vi "Set Double.vi"(8 "error in":errorcluster, 9 "value":dbl, 10 "variable name":string, 11 "GOLPI ref. in":T1={"pipe handle"={"lv_proc.dll file path"=path "", "process instance handle"=[], "debug mode"=FALSE, "debug data"=[]}, "fast read timeout [ms]"=500, "fast read settle time [ms]"=10, "fast read to multiple [ms]"=1, "max elements per input line"=100, "slow read timeout [ms]"=5000, "stdin double format specifier"="", "max elements per stdout output column"=100, "console mode bitstream"=FALSE, "bitstream first read timeout [ms]"=1000, "bitstream read timeout [ms]"=50, "struct transfer possible"=FALSE, "matlab mode"=FALSE}) -> (0 "error out":errorcluster, 3 "GOLPI ref. out":T1={"pipe handle"={"lv_proc.dll file path"=path "", "process instance handle"=[], "debug mode"=FALSE, "debug data"=[]}, "fast read timeout [ms]"=500, "fast read settle time [ms]"=10, "fast read to multiple [ms]"=1, "max elements per input line"=100, "slow read timeout [ms]"=5000, "stdin double format specifier"="", "max elements per stdout output column"=100, "console mode bitstream"=FALSE, "bitstream first read timeout [ms]"=1000, "bitstream read timeout [ms]"=50, "struct transfer possible"=FALSE, "matlab mode"=FALSE})   [LabVIEW 2020, in "GOLPI library.lvlib"]
doc: "Part of polymorph Set Variable.vi"
uses:
  GOLPI library.lvlib
  GOLPI reference Type Def.ctl
  Pipe Handle.ctl
  LV Process library.lvlib
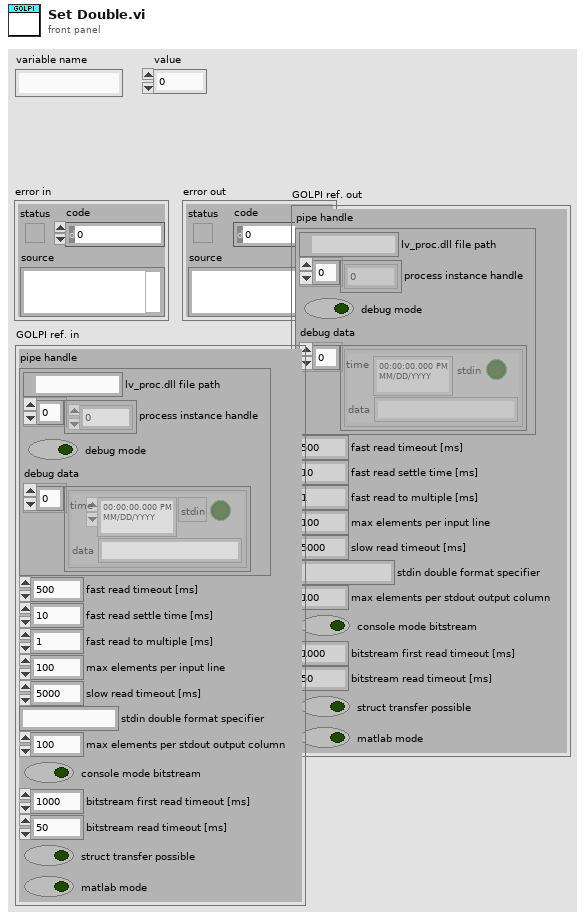
[diagram p1: front panel]
types:
  T1 = typedef "GOLPI library.lvlib/GOLPI reference Type Def.ctl" = cluster{"pipe handle":T2, "fast read timeout [ms]":u32, "fast read settle time [ms]":u32, "fast read to multiple [ms]":u32, "max elements per input line":u32, "slow read timeout [ms]":u32, "stdin double format specifier":string, "max elements per stdout output column":u32, "console mode bitstream":bool, "bitstream first read timeout [ms]":u32, "bitstream read timeout [ms]":u32, "struct transfer possible":bool, "matlab mode":bool}
  T2 = typedef "LV Process library.lvlib/Pipe Handle.ctl" = cluster{"lv_proc.dll file path":path, "process instance handle":u32[], "debug mode":bool, "debug data":cluster{"time":timestamp, "stdin":bool, "data":string}[]}
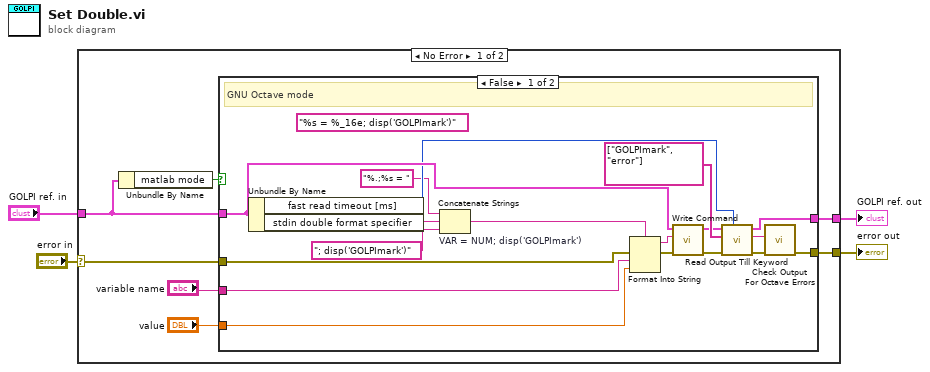
[diagram p0: block diagram]
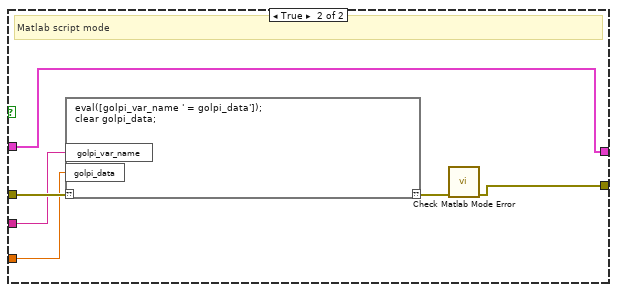
[diagram p2: hidden frame]
diagram:
  n1 = case shown="No Error" "error in" {
    selector: "error in" -> [w11 w37]
    tunnel: [w10 w37] -> w4
    tunnel: "GOLPI ref. in" -> [w8 w36]
    tunnel: [w9 w36] -> w1
    frame No Error {
      n2 = Unbundle By Name(w8) -> ("matlab mode"=w7:bool)
      n3 = case shown="False" w7 {
        tunnel: w11 -> [w29 w35]
        tunnel: [w21 w30] -> w10
        tunnel: [w20 w34] -> w9
        tunnel: w8 -> [w19 w34]
        tunnel: "variable name" -> [w13 w33]
        tunnel: "value" -> [w12 w32]
        frame False {
          (unwired) "%s = %_16e; disp('GOLPImark')" ("format string")
          # "GNU Octave mode"
          n4 = Unbundle By Name(w19) -> ("fast read timeout [ms]"=w18:u32, "stdin double format specifier"=w15:string)
          n5 = Concatenate Strings "VAR = NUM; disp('GOLPImark')"("%.;%s = " ("format string"), w15, "; disp('GOLPImark')" ("format string")) -> (w17:string)
          n6 = Format Into String(format string=w17, error in=w29, w13, w12) -> (resulting string=w27:string, error out=w28:errorcluster)  [unwired: 1 in]
          n7 = call "Write Command.vi"("error in"=w28, "command"=w27, "GOLPI ref. in"=w19) -> ("error out"=w26:errorcluster, "GOLPI ref. out"=w23:T1)  [unwired: 7 in]
          n8 = call "Read Output Till Keyword.vi"("timeout [ms]"=w18, "error in"=w26, "keywords"=string[] ["GOLPImark", "error"], "GOLPI ref. in"=w23) -> ("error out"=w25:errorcluster, "read buffer"=w22:string, "GOLPI ref. out"=w20:T1)  [unwired: 4 in, 1 out]
          n9 = call "Check Output For Octave Errors.vi"("error in"=w25, "read buffer"=w22) -> ("error out"=w21:errorcluster)  [unwired: 9 in]
        }
        frame True {
          # "Matlab script mode"
          n10 = script code="eval([golpi_var_name ' = golpi_data']);\nclear golpi_data;"("??"=w35, "golpi_data"=w32, "golpi_var_name"=w33) -> ("??"=w31:errorcluster)
          n11 = call "Check Matlab Mode Error.vi"("error in"=w31) -> ("error out"=w30:errorcluster)  [unwired: 10 in]
        }
      }
    }
    frame Error {
    }
  }
  "error out" <- w4
  "GOLPI ref. out" <- w1
